vi "ExcelFile_App.vi"(0 "읽기 경로":path=path "C:/Users/bsyim/Documents/LabVIEW Data/Vi_Code/Excel_File/Sample3_Worksheets_2.xlsx", 2 "Action(참)":bool=TRUE, 7 "File Name":string, 9 "Data(in)":string[][](array[string]), 11 "Work Sheet":i32=1, 12 "Read/Wirte(거짓:읽기)":bool) -> ()   [LabVIEW 2010]
panel:
  out "Data(out)":string[][](array[string])
  out "error out":errorcluster caption="에러 출력"
  in  "error in (no error)":errorcluster caption="에러 입력(에러 없음)"
  in  "정지":bool
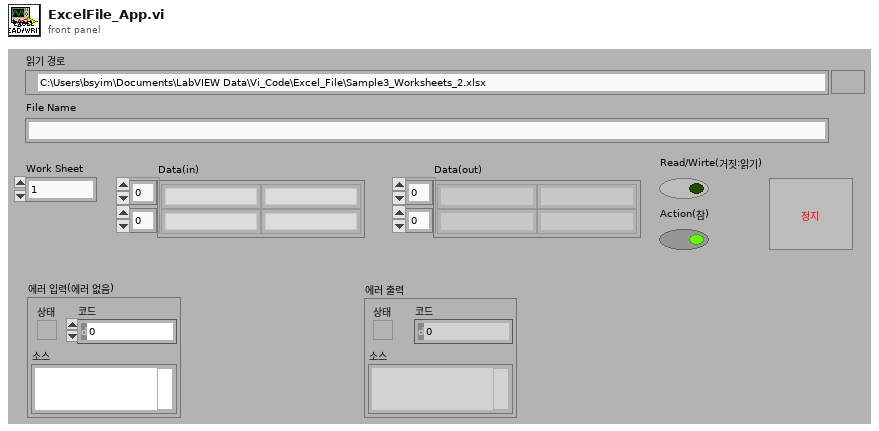
[diagram p1: front panel]
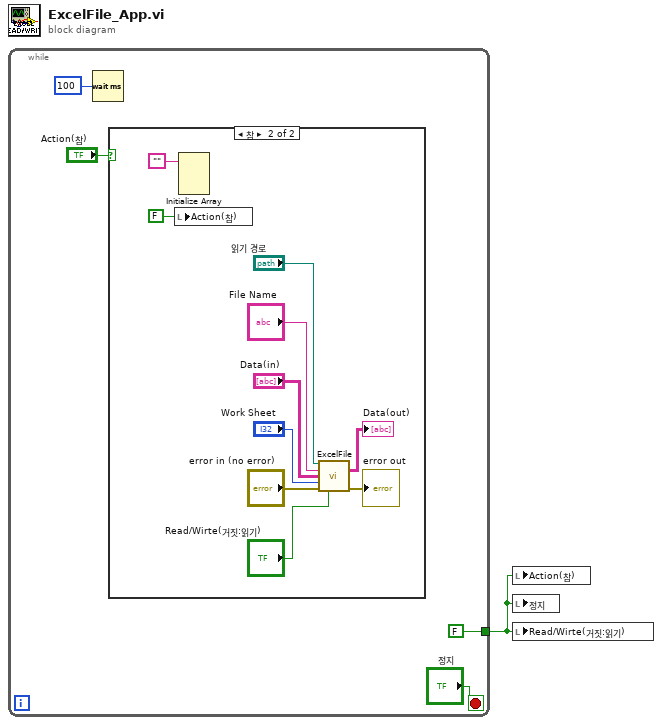
[diagram p0: block diagram]
diagram:
  n1 = while {
    tunnel: [FALSE] -> w1
    stop <- "정지" stop-if-true
    n2 = Wait (ms)(milliseconds to wait=u32 100) -> ()  [unwired: 1 out]
    n3 = case shown="참" "Action(참)" {
      frame False {
      }
      frame True {
        n4 = local write "Action(참)"(FALSE) -> ()
        n5 = Initialize Array("") -> ()  [unwired: 3 in, 1 out]
        n6 = call "ExcelFile.vi"("읽기 경로"="읽기 경로", "File Name"="File Name", "Data(in)"="Data(in)", "Work Sheet"="Work Sheet", "error in (no error)"="error in (no error)", "Read/Wirte(거짓:읽기)"="Read/Wirte(거짓:읽기)") -> ("2-D Data(out)"=→"Data(out)":string[][], "error out"=→"error out":errorcluster)  [unwired: 5 in, 3 out]
      }
    }
  }
  n7 = local write "Action(참)"(w1) -> ()
  n8 = local write "정지"(w1) -> ()
  n9 = local write "Read/Wirte(거짓:읽기)"(w1) -> ()
